vi "Do.vi"(8 "error in (no error)":errorcluster, 10 "Actor in":refnum<class "Actor.lvclass">, 11 "Update U8 Array":refnum<class "Update U8 Array.lvclass">) -> (0 "error out":errorcluster, 2 "Actor out":refnum<class "Actor.lvclass">)   [LabVIEW 2014, in "Update U8 Array.lvclass"]
doc: "(<B>Filename</B>: Actor Framework.lvlib:Message.lvclass:Do.vi)\n\nDefines what a message does when it is received by an actor. Generally, a message instructs an actor to invoke one of its methods. By default, this method does nothing. A child class must override it to define behavior. Create a child class by using the Actor Framework Message Maker dialog box."
uses:
  Update U8 Array.lvclass
  <vilib>/NI/Current Value Table/DataTypes/Array of U8_Write.vi
  <vilib>/ActorFramework/Actor/Actor.lvclass
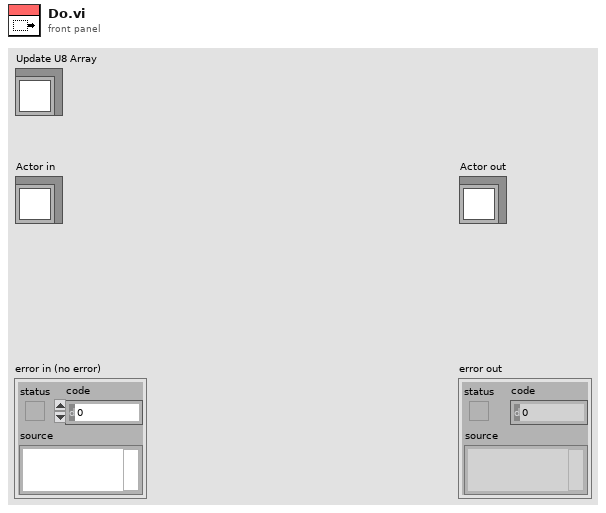
[diagram p1: front panel]
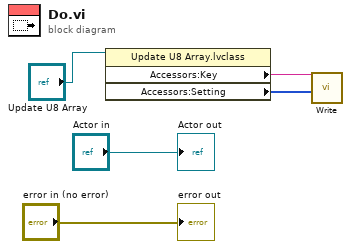
[diagram p0: block diagram]
diagram:
  n1 = property class="Update U8 Array.lvclass"(reference="Update U8 Array") -> ("Accessors:Key"=w2:string, "Accessors:Setting"=w1:u8[])  [unwired: 1 in, 2 out]
  n2 = call-poly <vilib>:"Write.vi"("Value"=w1, "Tag Name"=w2) -> ()  [unwired: 9 in, 1 out]
  "error out" <- "error in (no error)"
  "Actor out" <- "Actor in"
